vi "read Booleans.vi"(10 "indices":i32[](array[numeric]), 11 "data table in":T1) -> (1 "values":bool[](array[boolean]), 3 "data table out":T1)   [LabVIEW 2013, in "data bus values.lvlib"]
doc: "Reads a set of values from the data table. Requires an index for every value."
uses:
  data bus values.lvlib
  data table.ctl
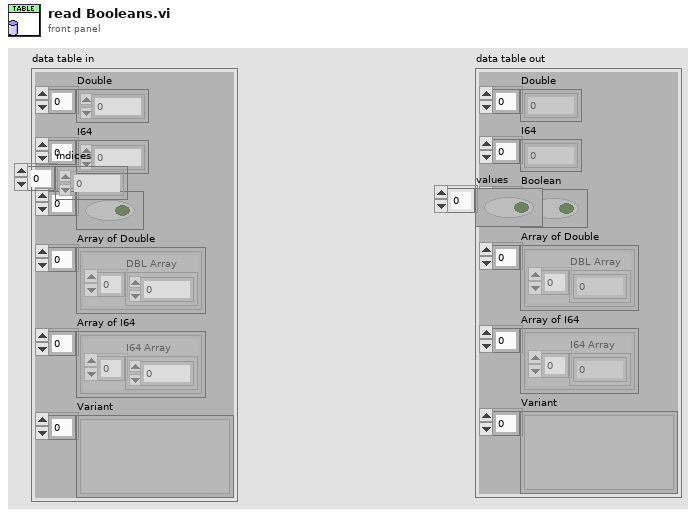
[diagram p1: front panel]
types:
  T1 = typedef "data bus values.lvlib/data table.ctl" = cluster{"Double":dbl[], "I64":i64[], "Boolean":bool[], "Array of Double":cluster{"DBL Array":dbl[]}[], "Array of I64":cluster{"I64 Array":i64[]}[], "Variant":variant[]}
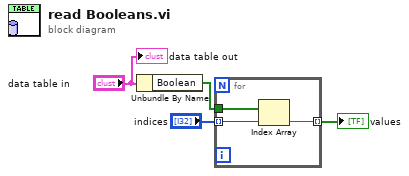
[diagram p0: block diagram]
diagram:
  n1 = Unbundle By Name("data table in") -> ("Boolean"=w3:bool[])
  n2 = for {
    tunnel: w3 -> [w7]
    tunnel: [w6] -> w2 mode=indexing
    tunnel: "indices" -> [w5] mode=indexing
    n3 = Index Array(array=w7, index=w5) -> (element=w6:bool)
  }
  "values" <- w2
  "data table out" <- "data table in"
